vi "Setup UI.vi"(8 "error in (no error)":errorcluster, 10 "Set UI to input? (F)":bool, 11 "Microwave Freq Scan in":refnum<class "Microwave Freq Scan.lvclass">) -> (0 "error out":errorcluster, 3 "Microwave Freq Scan out":refnum<class "Microwave Freq Scan.lvclass">)   [LabVIEW 2015, in "Microwave Freq Scan.lvclass"]
doc: "Scanner::Setup is a constructor that has no parameters and faces the user. The Factory calls this VI to let the user configure this Scanner. It is dynamically dispatched in order to let the user choose the type as well as the options of the scanner."
uses:
  Microwave Freq Scan.lvclass
  Microwave Freq Scan.lvclass/Microwave Freq Scan.ctl
  Instruments/Utility Classes/Scannable/Scannable.lvclass
  Instruments/Microwave/Agilent PSG MXG Series/Agilent PSG MXG Series.lvlib
panel:
  in  "rf on/off":bool
  in  "Send conds for \nfirst point to MW Gen":bool
  in  "Amplitude (dBm)":dbl
  # "Microwave Freq Scan"
  # "Note: Independent variable \nabove must be given in GHz"
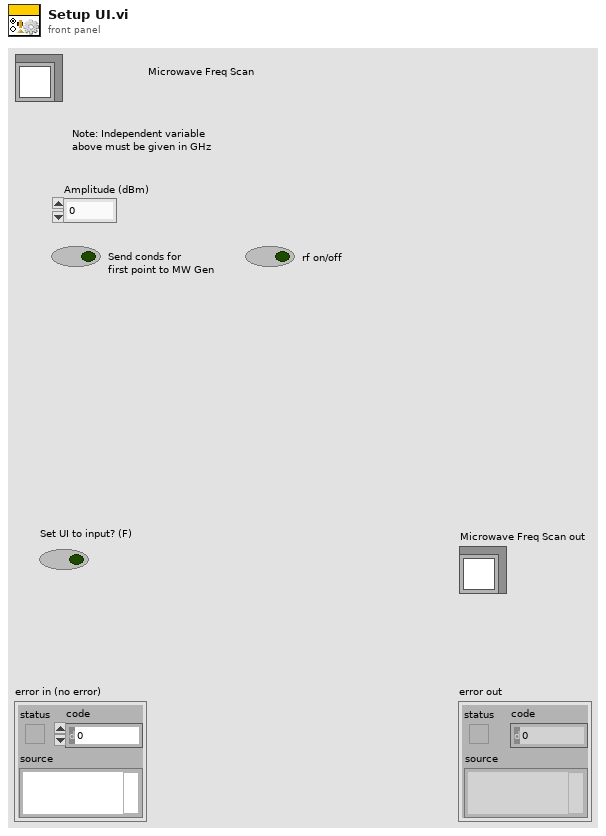
[diagram p1: front panel]
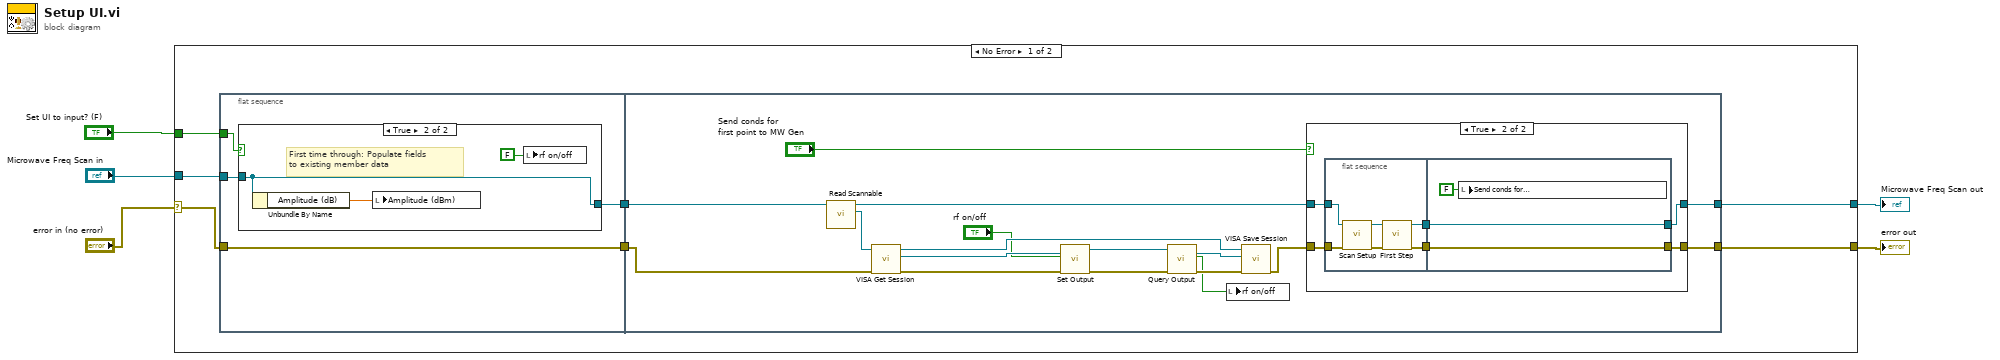
[diagram p0: block diagram]
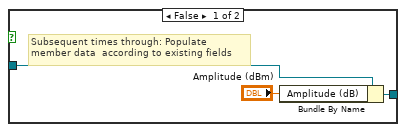
[diagram p2: hidden frame]
diagram:
  n1 = case shown="No Error" "error in (no error)" {
    selector: "error in (no error)" -> [w6 w57]
    tunnel: "Set UI to input? (F)" -> [w10 _]
    tunnel: [w9 w58] -> w4
    tunnel: [w8 w57] -> w3
    tunnel: "Microwave Freq Scan in" -> [w7 w58]
    frame No Error {
      n2 = flat-sequence {
        tunnel: w10 -> [w16]
        tunnel: [w15] -> w12
        tunnel: w7 -> [w14]
        tunnel: w6 -> [w13]
        tunnel: [w13] -> w11
        tunnel: w12 -> [w36]
        tunnel: [w38] -> w9
        tunnel: [w37] -> w8
        tunnel: w11 -> [w28]
        frame #0 {
          n3 = case shown="True" w16 {
            tunnel: [w18 w22] -> w15
            tunnel: w14 -> [w19 w22]
            frame False {
              # "Subsequent times through: Populate \nmember data  according to existing fields"
              n4 = Bundle By Name(cluster=w19, "Amplitude (dB)"="Amplitude (dBm)") -> (w18:refnum<class "Microwave Freq Scan.lvclass">)
            }
            frame True {
              # "First time through: Populate fields  \nto existing member data"
              n5 = Unbundle By Name(w22) -> ("Amplitude (dB)"=w21:dbl)
              n6 = local write "Amplitude (dBm)"(w21) -> ()
              n7 = local write "rf on/off"(FALSE ("rf on/off")) -> ()
            }
          }
        }
        frame #1 {
          n8 = call-dynamic "Read Scannable.vi"("Scanner.lvclass in"=w36) -> ("Scannable.lvclass"=w34:refnum<class "Scannable.lvclass">, "Scanner.lvclass out"=w35:refnum<class "Microwave Freq Scan.lvclass">)  [unwired: 1 in, 8 out]
          n9 = call-dynamic "VISA Get Session.vi"("error in (no error)"=w28, "Instrument.lvclass in"=w34) -> ("error out"=w27:errorcluster, "VISA Resource Name"=w33:refnum<visa-resource-name>, "Instrument.lvclass out"=w32:refnum<class "Scannable.lvclass">)  [unwired: 7 out]
          n10 = call "Set Output.vi"("error in (no error)"=w27, "Output On"="rf on/off", "VISA resource name"=w33) -> ("error out"=w26:errorcluster, "VISA resource name out"=w31:refnum<visa-resource-name>)  [unwired: 7 out]
          n11 = call "Query Output.vi"("error in (no error)"=w26, "VISA resource name"=w31) -> ("error out"=w25:errorcluster, "Output On?"=w23:bool, "VISA resource name out"=w30:refnum<visa-resource-name>)  [unwired: 7 out]
          n12 = local write "rf on/off"(w23) -> ()
          n13 = call-dynamic "VISA Save Session.vi"("error in (no error)"=w25, "VISA Resource Name"=w30, "Instrument.lvclass in"=w32) -> ("error out"=w24:errorcluster)  [unwired: 8 out]
          n14 = case shown="True" "Send conds for \nfirst point to MW Gen" {
            tunnel: w35 -> [w41 w47]
            tunnel: [w41 w46] -> w38
            tunnel: [w40 w45] -> w37
            tunnel: w24 -> [w40 w44]
            frame False {
            }
            frame True {
              n15 = flat-sequence {
                tunnel: w47 -> [w51]
                tunnel: w44 -> [w48]
                tunnel: [w50] -> w43
                tunnel: [w49] -> w42
                tunnel: [w55] -> w45
                tunnel: [w56] -> w46
                tunnel: w43 -> [w56]
                tunnel: w42 -> [w55]
                frame #0 {
                  n16 = call-dynamic "Scan Setup.vi"("error in (no error)"=w48, "Microwave Freq Scan in"=w51) -> ("error out"=w52:errorcluster, "Microwave Freq Scan out"=w53:refnum<class "Microwave Freq Scan.lvclass">)  [unwired: 8 out]
                  n17 = call-dynamic "First Step.vi"("error in (no error)"=w52, "Microwave Freq Scan.lvclass in"=w53) -> ("error out"=w49:errorcluster, "Microwave Freq Scan.lvclass out"=w50:refnum<class "Microwave Freq Scan.lvclass">)  [unwired: 8 out]
                }
                frame #1 {
                  n18 = local write "Send conds for \nfirst point to MW Gen"(FALSE ("Send conds for first point to MW Gen")) -> ()
                }
              }
            }
          }
        }
      }
    }
    frame Error {
    }
  }
  "error out" <- w3
  "Microwave Freq Scan out" <- w4
